vi "PV HLT5xx Physical units.vi"(6 "set pressure":u16(ring) items=["mbar", "Pa", "Atm", "Torr"], 7 "Adress of unit":u16=1 min=1 max=999 step=1, 8 "error in (no error)":errorcluster, 9 "set leakrate":u16(ring) items=["mbar l/s", "Pam3 /s", "Atm cc/s", "Torr l/s", "sccm", "sccs", "ppm", "g / a", "oz / yr"], 10 "Parameter\nread only<->describe":bool, 11 "VISA session":refnum<visa-resource-name>) -> (0 "error out":errorcluster, 1 "leakrate out":u16(ring) items=["mbar l/s", "Pam3 /s", "Atm cc/s", "Torr l/s", "sccm", "sccs", "ppm", "g / a", "oz / yr"], 2 "response (data)":string, 3 "dup VISA session":refnum<visa-resource-name>, 4 "pressure out":u16(ring) items=["mbar", "Pa", "Atm", "Torr"])   [LabVIEW 2016, in "Pfeiffer Vacuum.lvlib"]
doc: "This VI allows you to set or check the \"Physical units (Para 643)\" on the SmartTest (HLT5xx)."
uses:
  Pfeiffer Vacuum.lvlib
panel:
  # "Physical units"
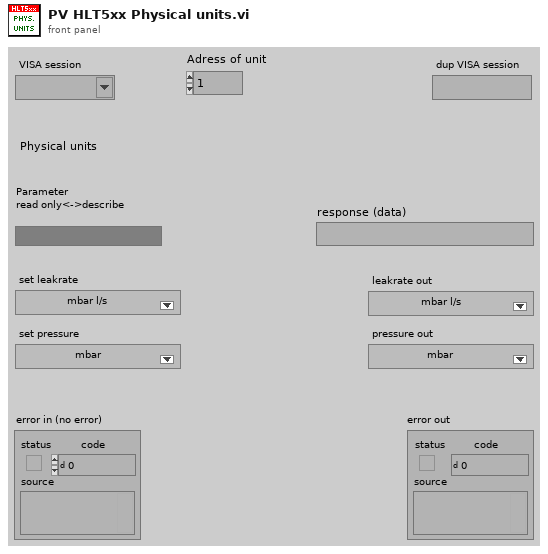
[diagram p1: front panel]
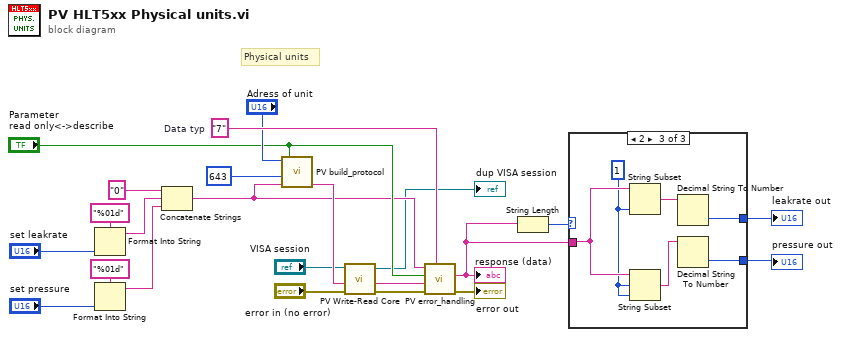
[diagram p0: block diagram]
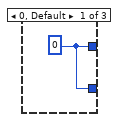
[diagram p2: hidden frame]
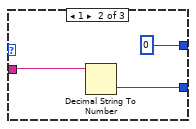
[diagram p3: hidden frame]
diagram:
  w19 = "7"  # Data typ
  # "Physical units"
  n1 = Format Into String(format string="%01d" ("Format-String"), "set leakrate") -> (resulting string=w10:string)  [unwired: 2 in, 1 out]
  n2 = Format Into String(format string="%01d" ("Format-String"), "set pressure") -> (resulting string=w9:string)  [unwired: 2 in, 1 out]
  n3 = Concatenate Strings("0" ("Resultierender String"), w10, w9) -> (w8:string)
  n4 = call "PV build_protocol.vi"("Data"=w8, "Parameter-number"=u16 643, "parameter\nread<->describe"="Parameter\nread only<->describe", "Adress"="Adress of unit") -> ("output"=w22:string)  [unwired: 3 in]
  n5 = call "PV Write-Read Core.vi"("error in"="error in (no error)", "Write data in"=w22, "VISA session"="VISA session") -> ("error out"=w20:errorcluster, "response (data) out"=w21:string, "dup VISA session"=→"dup VISA session":refnum<visa-resource-name>)  [unwired: 2 in]
  n6 = call "PV error_handling.vi"("Data Typ in"=w19, "error in"=w20, "response (data) in"=w21, "Parameter\nread only<->describe"="Parameter\nread only<->describe", "data in"=w8) -> ("error out"=→"error out":errorcluster, "Data out"=w4:string)  [unwired: 4 in, 1 out]
  "response (data)" <- w4
  n7 = String Length(string=w4) -> (length=w5:i32)
  n8 = case shown="2" w5 {
    tunnel: w4 -> [_ w27 w31]
    tunnel: [w24 0 w32] -> w2
    tunnel: [w24 w25 w33] -> w3
    frame 0, Default {
      w24 = 0
    }
    frame 1 {
      n9 = Decimal String To Number(string=w27) -> (number=w25:i32)  [unwired: 2 in, 1 out]
    }
    frame 2 {
      w28 = 1
      n10 = String Subset(string=w31, length (rest)=w28) -> (substring=w30:string)  [unwired: 1 in]
      n11 = String Subset(string=w31, offset (0)=w28, length (rest)=w28) -> (substring=w29:string)
      n12 = Decimal String To Number(string=w30) -> (number=w32:i32)  [unwired: 2 in, 1 out]
      n13 = Decimal String To Number(string=w29) -> (number=w33:i32)  [unwired: 2 in, 1 out]
    }
  }
  "leakrate out" <- w2
  "pressure out" <- w3
